vi "tipdefinition 1point.vi"(5 "radius of curvature":dbl min=-0.0 max=1000.0 format="%.2f", 7 "x":dbl, 9 "tipangle":dbl=1.0 min=1.0 max=89.0 format="%.2f", 11 "offset":i32=1) -> (4 "result":dbl)   [LabVIEW 2017]
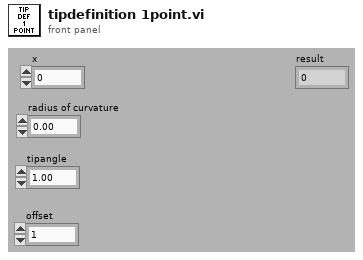
[diagram p1: front panel]
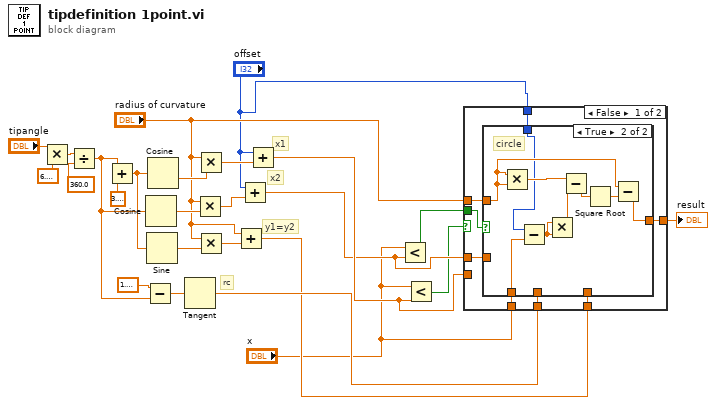
[diagram p0: block diagram]
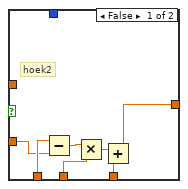
[diagram p2: hidden frame]
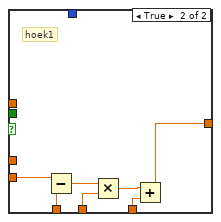
[diagram p3: hidden frame]
diagram:
  # "rc"
  # "y1=y2"
  # "x2"
  # "x1"
  n1 = Multiply(x="tipangle", y=6.283185307179586) -> (x*y=w23:dbl)
  n2 = Divide(x=w23, y=360.0) -> (x/y=w12:dbl)
  n3 = Add(x=w12, y=3.141592653589793) -> (x+y=w16:dbl)
  n4 = Subtract(x=1.5707963267948966, y=w12) -> (x-y=w11:dbl)
  n5 = Cosine(x=w12) -> (cos(x)=w19:dbl)
  n6 = Sine(x=w16) -> (sin(x)=w15:dbl)
  n7 = Cosine(x=w16) -> (cos(x)=w20:dbl)
  n8 = Tangent(1:w11) -> (0:w8:dbl)
  n9 = Multiply(x="radius of curvature", y=w19) -> (x*y=w18:dbl)
  n10 = Multiply(x="radius of curvature", y=w20) -> (x*y=w17:dbl)
  n11 = Multiply(x="radius of curvature", y=w15) -> (x*y=w14:dbl)
  n12 = Add(x="radius of curvature", y=w14) -> (x+y=w7:dbl)
  n13 = Add(x="offset", y=w18) -> (x+y=w9:dbl)
  n14 = Add(x="offset", y=w17) -> (x+y=w10:dbl)
  n15 = Less?(x="x", y=w9) -> (x < y?=w2:bool)
  n16 = Less?(x="x", y=w10) -> (x < y?=w3:bool)
  n17 = case shown="False" w3 {
    tunnel: w10 -> [_ w56]
    tunnel: "x" -> [w32 w55]
    tunnel: w8 -> [w31 w53]
    tunnel: [w29 w50] -> w5
    tunnel: w9 -> [w33 _]
    tunnel: w7 -> [w30 w52]
    tunnel: w2 -> [w28 _]
    tunnel: "radius of curvature" -> [w27 _]
    tunnel: "offset" -> [w26 _]
    frame False {
      n18 = case shown="True" w28 {
        tunnel: w33 -> [w39 _]
        tunnel: w32 -> [w40 w49]
        tunnel: w31 -> [w37 _]
        tunnel: w30 -> [w35 _]
        tunnel: [w34 w42] -> w29
        tunnel: w27 -> [_ w43]
        tunnel: w26 -> [_ w41]
        frame False {
          # "hoek2"
          n19 = Subtract(x=w40, y=w39) -> (x-y=w38:dbl)
          n20 = Multiply(x=w38, y=w37) -> (x*y=w36:dbl)
          n21 = Add(x=w36, y=w35) -> (x+y=w34:dbl)
        }
        frame True {
          # "circle"
          n22 = Multiply(x=w43, y=w43) -> (x*y=w48:dbl)
          n23 = Subtract(x=w41, y=w49) -> (x-y=w47:dbl)
          n24 = Multiply(x=w47, y=w47) -> (x*y=w46:dbl)
          n25 = Subtract(x=w48, y=w46) -> (x-y=w45:dbl)
          n26 = Square Root(x=w45) -> (sqrt(x)=w44:dbl)
          n27 = Subtract(x=w43, y=w44) -> (x-y=w42:dbl)
        }
      }
    }
    frame True {
      # "hoek1"
      n28 = Subtract(x=w56, y=w55) -> (x-y=w54:dbl)
      n29 = Multiply(x=w54, y=w53) -> (x*y=w51:dbl)
      n30 = Add(x=w51, y=w52) -> (x+y=w50:dbl)
    }
  }
  "result" <- w5
